vi "Register Auto-Events.vi"(8 "error in (no error)":errorcluster, 10 "Controls":T2, 11 "VI":refnum<vi>) -> (0 "error out":errorcluster, 2 "Stop!":refnum<user-event>, 3 "Auto-Event Registration Refnum":T1)   [LabVIEW 2017, in "AutoRegistration.lvlib" / "AutoRegistration.lvclass"]
doc: "<License>\nCopyright © 2017 Composed Systems, LLC | All rights reserved\nwww.composed.io\n\nAuthor: Ethan Stern <ethan.stern@composed.io>\n\nThis software is provided \"AS IS\" WITHOUT WARRANTIES, either express or implied, AND IS FOR EDUCATIONAL PURPOSES ONLY.\n</License>"
uses:
  AutoRegistration.lvclass
  Registration References.ctl
  Auto-Event Registration Refnum.ctl
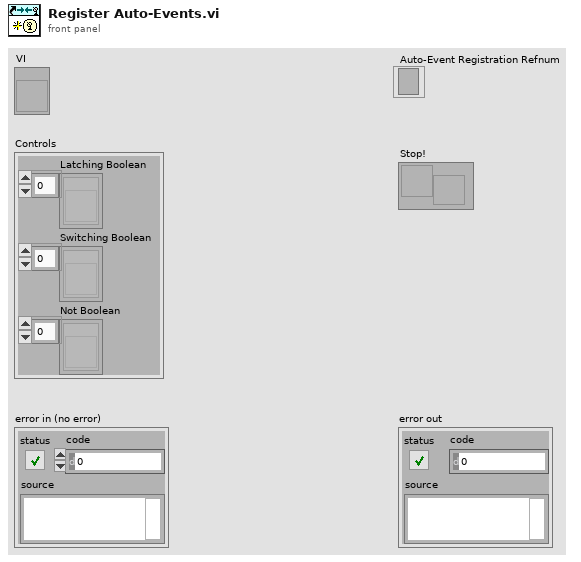
[diagram p1: front panel]
types:
  T1 = typedef "AutoRegistration.lvlib/AutoRegistration.lvclass/Auto-Event Registration Refnum.ctl" = refnum<event-registration>
  T2 = typedef "AutoRegistration.lvlib/AutoRegistration.lvclass/Registration References.ctl" = cluster{"Latching Boolean":refnum<vi>[], "Switching Boolean":refnum<vi>[], "Not Boolean":refnum<vi>[]}
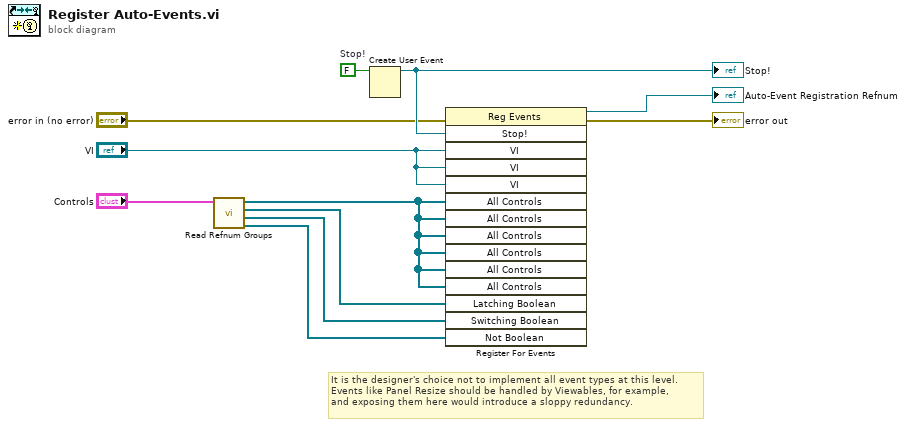
[diagram p0: block diagram]
diagram:
  w10 = FALSE  # Stop!
  # "It is the designer's choice not to implement all event types at this level.\nEvents like Panel Resize should be handled by Viewables, for example,\nand exposing them here would introduce a sloppy redundancy."
  n1 = call "Read Refnum Groups.vi"("All Controls in"="Controls") -> ("Not Boolean"=w3:refnum<vi>[], "Switching Boolean"=w4:refnum<vi>[], "Latching Boolean"=w5:refnum<vi>[], "All Controls"=w2:refnum<vi>[])  [unwired: 7 in]
  n2 = Create User Event(user event datatype=w10) -> (user event=w11:refnum<user-event>)  [unwired: 1 in, 1 out]
  "Stop!" <- w11
  n3 = register-events(error in="error in (no error)", w11, "VI", "VI", "VI", w2, w2, w2, w2, w2, w2, w5, w4, w3) -> (reference out=→"Auto-Event Registration Refnum":refnum<event-registration>, error out=→"error out":errorcluster)  [unwired: 1 in]
